vi "GetHardwareListing.vi"() -> (0 "Devices":path[](array[path]), 1 "Array":string[](array[string]))   [LabVIEW 2014]
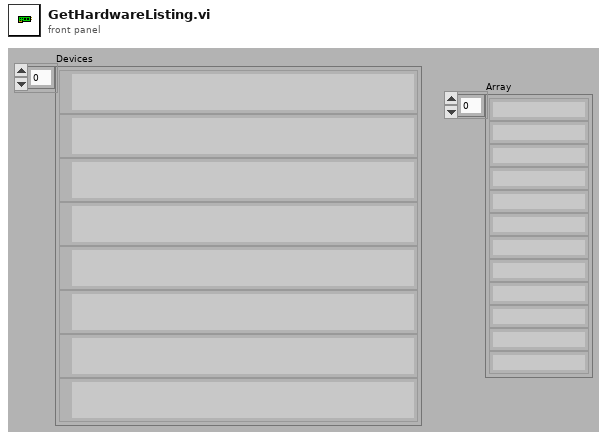
[diagram p1: front panel]
types:
  T1 = typedef "BotSpeak.HardwareSpecs.ctl" = cluster{"Hardware Name":string, "Hardware URL":string, "ComType":enum16{"Undefined", "HTTP", "Serial", "TCPIP", "Console"}, "TCP Port":i32, "DefaultAddress":string, "Retries":i32, "Translate":enum16{"None", "Tiny", "URAPI"}, "MaxScriptSize":i32, "MaxVarNumber":i32, "StartupWait":i32, "Patience":i32, "Startup Patience":i32, "Hardware Help":string, "Com Protocol":string, "Translator":cluster{"BotSpeak CMD":string, "CMD out":string}[], "Init Code":string, "Variable Format":enum16{"INT", "FLOAT", "FIXED"}, "username":string, "password":string}
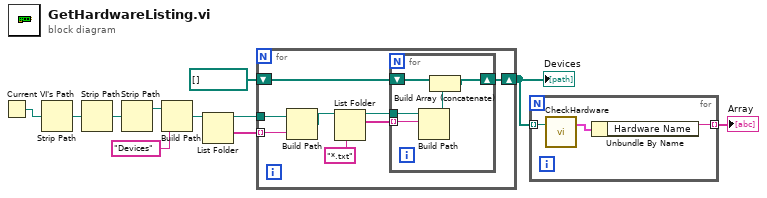
[diagram p0: block diagram]
diagram:
  n1 = Current VI's Path() -> (path=w11:path)
  n2 = Strip Path(path=w11) -> (stripped path=w10:path)  [unwired: 1 out]
  n3 = Strip Path(path=w10) -> (stripped path=w9:path)  [unwired: 1 out]
  n4 = Strip Path(path=w9) -> (stripped path=w8:path)  [unwired: 1 out]
  n5 = Build Path(base path=w8, name or relative path="Devices") -> (appended path=w6:path)
  n6 = List Folder(path=w6) -> (path out=w4:path, folder names=w5:string[])  [unwired: 3 in, 2 out]
  n7 = for {
    tunnel: w5 -> [w19] mode=indexing
    tunnel: w4 -> [w18]
    shift-right: [w12] -> w2
    shift-left: path[] [] -> [w13]
    n8 = Build Path(base path=w18, name or relative path=w19) -> (appended path=w17:path)
    n9 = List Folder(path=w17, pattern="*.txt") -> (path out=w15:path, filenames=w14:string[])  [unwired: 2 in, 2 out]
    n10 = for {
      tunnel: w15 -> [w24]
      tunnel: w14 -> [w23] mode=indexing
      shift-right: [w22] -> w12
      shift-left: w13 -> [w21]
      n11 = Build Path(base path=w24, name or relative path=w23) -> (appended path=w20:path)
      n12 = Build Array (concatenate)(w21, w20) -> (w22:path[])
    }
  }
  "Devices" <- w2
  n13 = for {
    tunnel: w2 -> [w27] mode=indexing
    tunnel: [w25] -> w1 mode=indexing
    n14 = call <userlib>:"CheckHardware.vi"("Hardware"=w27) -> ("HardwareSpecs"=w26:T1)  [unwired: 2 in]
    n15 = Unbundle By Name(w26) -> ("Hardware Name"=w25:string)
  }
  "Array" <- w1
